vi "clear Session Data.vi"(0 "Session in":refnum<class "niRFSTS Sequence Flow.lvclass">, 11 "error in":errorcluster) -> (4 "Session out":refnum<class "niRFSTS Sequence Flow.lvclass">, 15 "error out":errorcluster)   [LabVIEW 2018, in "niRFSTS Sequence Flow.lvclass"]
uses:
  niRFSTS Sequence Flow.lvclass
  niRFSTS Sequence Flow.lvclass/niRFSTS Sequence Flow.ctl
  Plugins/Measurement Interface.lvlibp/Measurement Interface.lvclass
  Plugins/Sequence Automation Session.lvlibp/Sequence Automation Session.lvclass
  Plugins/TestStand API Tools (TSAT).lvlibp/Sequence File Actions/TSAT Sequence File Actions.lvlib
  Plugins/Test Number and Bin Generator.lvlibp/Test Number and Bin Generator/Test Number and Bin Generator.lvclass
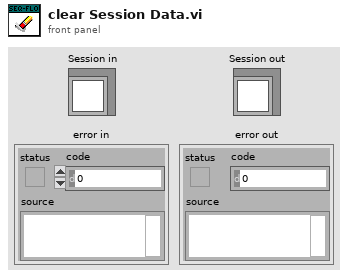
[diagram p1: front panel]
types:
  T1 = typedef "Test Number and Bin Generator.lvlibp/Test Number and Bin Generator.lvclass/Session Handle.ctl" = refnum<data-value>
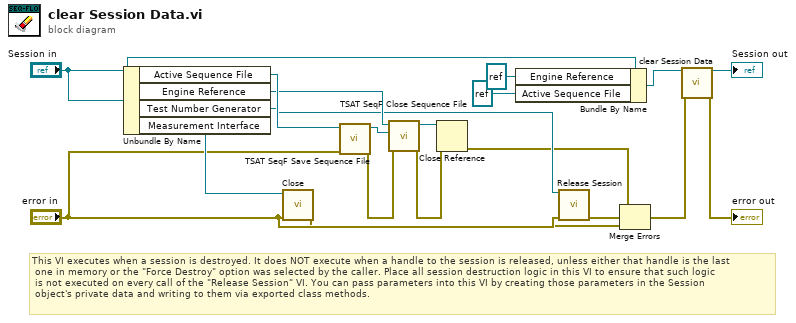
[diagram p0: block diagram]
diagram:
  # "This VI executes when a session is destroyed. It does NOT execute when a handle to the session is released, unless either that handle is the last\n one in memory or the \"Force Destroy\" option was selected by the caller. Place all session destruction logic in this VI to ensure that such logic\n is not executed on every call of the \"Release Session\" VI. You can pass parameters into this VI by creating those parameters in the Session \n object's private data and writing to them via exported class methods."
  n1 = Unbundle By Name("Session in") -> ("Active Sequence File"=w15:refnum<k7>, "Engine Reference"=w14:refnum<k7>, "Test Number Generator"=w6:T1, "Measurement Interface"=w5:refnum<class "Measurement Interface.lvclass">)
  n2 = call-dynamic "Close.vi"("error in (no error)"="error in", "Measurement Interface in"=w5) -> ("error out"=w1:errorcluster)  [unwired: 8 in, 1 out]
  n3 = call "TSAT SeqF Save Sequence File.vi"("Error in"="error in", "Sequence File In"=w15) -> ("Error out"=w17:errorcluster, "Sequence File Out"=w13:refnum<k7>)  [unwired: 8 in]
  n4 = call "TSAT SeqF Close Sequence File.vi"("Error In"=w17, "Sequence File In"=w13, "Engine In"=w14) -> ("Error Out"=w16:errorcluster, "Engine out"=w12:refnum<k7>)  [unwired: 7 in]
  n5 = Close Reference(reference=w12, error in (no error)=w16) -> (error out=w2:errorcluster)
  n6 = Bundle By Name(cluster="Session in", "Engine Reference"=refnum<k7> refnum, "Active Sequence File"=refnum<k7> refnum) -> (w8:refnum<class "niRFSTS Sequence Flow.lvclass">)
  n7 = call "Release Session.vi"("Session Handle"=w6, "error in (no error)"="error in") -> ("error out"=w7:errorcluster)  [unwired: 13 in]
  n8 = Merge Errors(w2, w7, w1) -> (w3:errorcluster)
  n9 = call-parent "clear Session Data.vi"("OBJ - Measurement Session in"=w8, "error in"=w3) -> ("OBJ - Measurement Session out"=→"Session out":refnum<class "niRFSTS Sequence Flow.lvclass">, "error out"=→"error out":errorcluster)  [unwired: 12 in]
